vi "Log Field (No Objects).vi"(8 "error in (no error)":errorcluster, 11 "Cluster In":T4={"Field"=0.0, "Rate"=0.0, "Status"={"Sweeping"=FALSE, "Clamped"=FALSE, "Hold"=FALSE, "At Rest"=FALSE, "Quench"=FALSE, "Persistent Mode"=FALSE, "Switch Heater"=FALSE}, "ILM Shut Down?"=FALSE, "IO Info"={"Address"={"Com Port"=1, "ISOBUS Address"=2, "GPIB Address"=24, "Communication"=enum."ISOBUS"}, "Version"=enum."IPS"}, "IO Info (Level Meter)"={"Address"={"Com Port"=1, "ISOBUS Address"=5, "GPIB Address"=24, "Communication"=enum."ISOBUS"}, "ILM Name"="", "Display Channel"=[]}, "Training?"=FALSE, "Training Field and Speed Cluster"={"Training Field"=[0.0, 4.108, 5.78, 8.001], "Training Speed"=[0.0057, 0.0022833333333333334, 0.0011333333333333334, 0.0011333333333333334]}}) -> (0 "error out":errorcluster, 3 "Cluster Out":T4={"Field"=0.0, "Rate"=0.0, "Status"={"Sweeping"=FALSE, "Clamped"=FALSE, "Hold"=FALSE, "At Rest"=FALSE, "Quench"=FALSE, "Persistent Mode"=FALSE, "Switch Heater"=FALSE}, "ILM Shut Down?"=FALSE, "IO Info"={"Address"={"Com Port"=1, "ISOBUS Address"=2, "GPIB Address"=24, "Communication"=enum."ISOBUS"}, "Version"=enum."IPS"}, "IO Info (Level Meter)"={"Address"={"Com Port"=1, "ISOBUS Address"=5, "GPIB Address"=24, "Communication"=enum."ISOBUS"}, "ILM Name"="", "Display Channel"=[]}, "Training?"=FALSE, "Training Field and Speed Cluster"={"Training Field"=[0.0, 4.108, 5.78, 8.001], "Training Speed"=[0.0057, 0.0022833333333333334, 0.0011333333333333334, 0.0011333333333333334]}})   [LabVIEW 2009]
uses:
  Magnet status.ctl
  Oxford/PSSUBS.LLB/PSIO.ctl
  Oxford/BUSGEN.LLB/OxfordAddress.ctl
  Global/File Locations.vi
  Power Supply.lvclass
panel:
  out "Field":dbl[unit]
  out "status":string
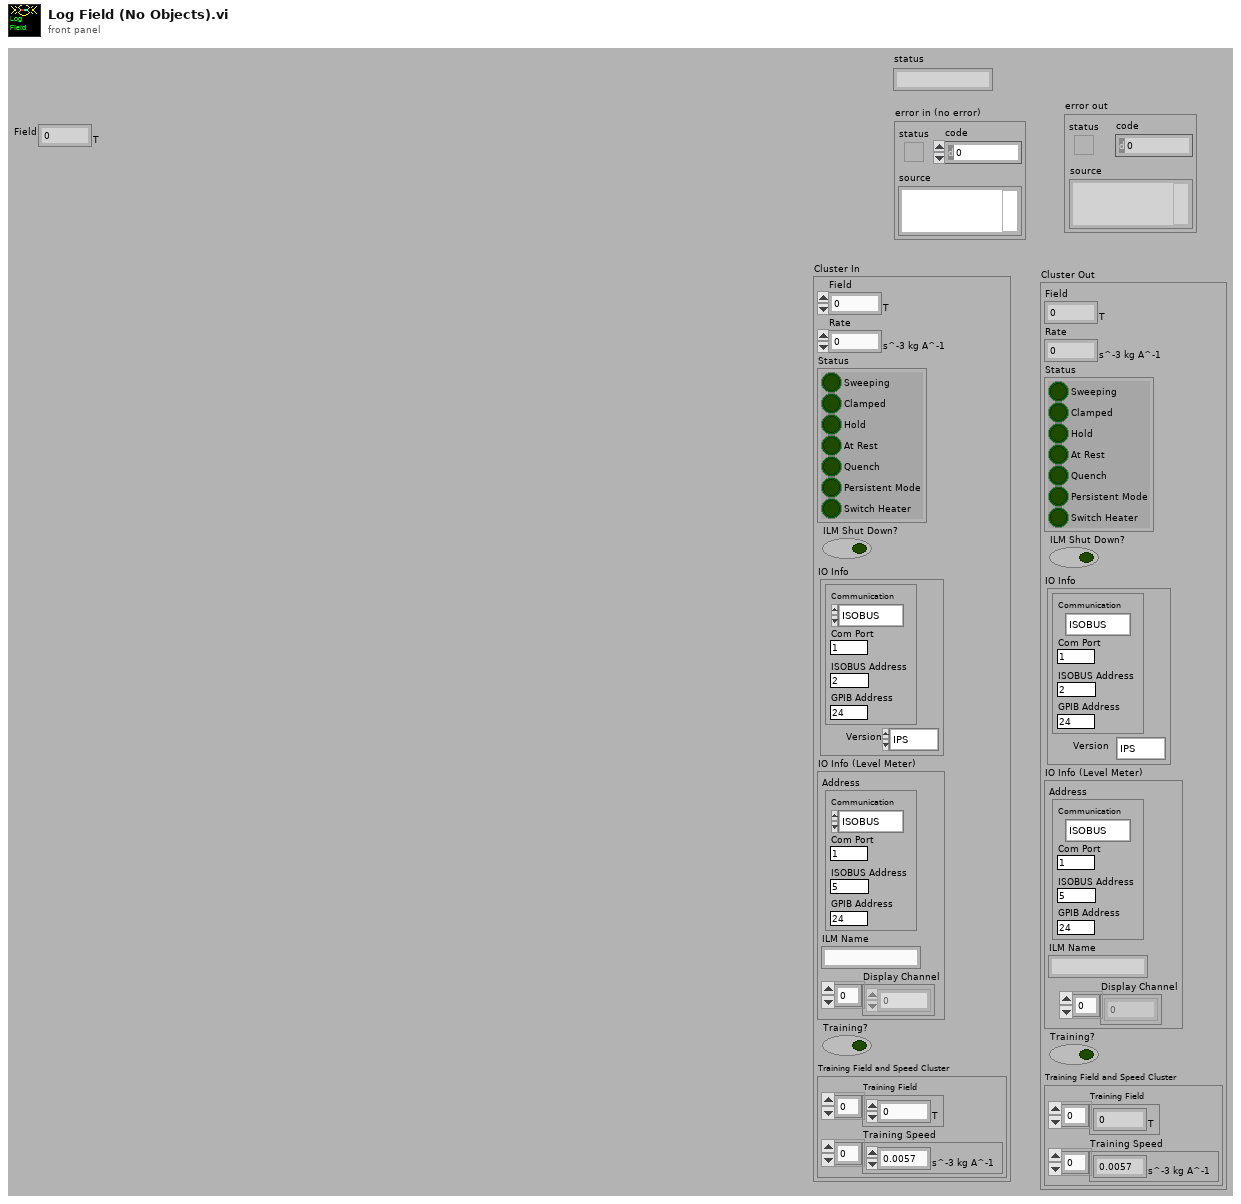
[diagram p1: front panel]
types:
  T1 = typedef "Power Supply.lvclass/Magnet status.ctl" = cluster{"Sweeping":bool, "Clamped":bool, "Hold":bool, "At Rest":bool, "Quench":bool, "Persistent Mode":bool, "Switch Heater":bool}
  T2 = typedef "PSIO.ctl" = cluster{"Address":T3, "Version":enum16{"PS", "IPS"}}
  T3 = typedef "OxfordAddress.ctl" = cluster{"Com Port":i32, "ISOBUS Address":i32, "GPIB Address":i16, "Communication":enum16{"RS232", "ISOBUS", "GPIB", "Gateway"}}
  T4 = cluster{"Field":dbl[unit], "Rate":dbl[unit], "Status":T1, "ILM Shut Down?":bool, "IO Info":T2, "IO Info (Level Meter)":cluster{"Address":T3, "ILM Name":string, "Display Channel":i32[]}, "Training?":bool, "Training Field and Speed Cluster":cluster{"Training Field":dbl[unit][], "Training Speed":dbl[unit][]}}
  T5 = enum16{"open", "open or create", "create or replace", "create", "open (read only)"}
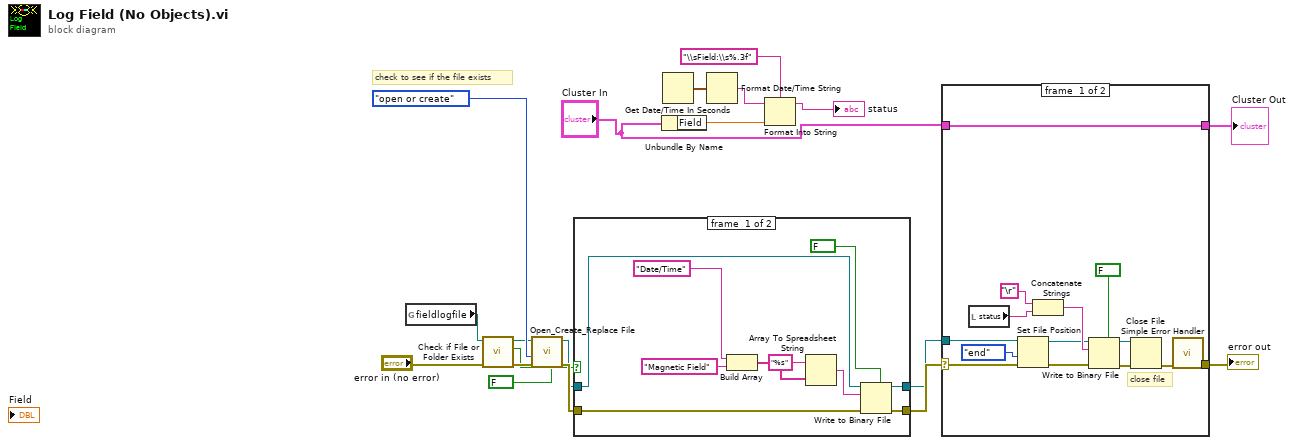
[diagram p0: block diagram]
diagram:
  # "check to see if the file exists"
  n1 = global read "File Locations.vi" "fieldlogfile"() -> (w10:path)
  n2 = call <vilib>:"Check if File or Folder Exists.vi"("error in (no error)"="error in (no error)", "path"=w10) -> ("error out"=w18:errorcluster, "file or folder exists?"=w14:bool, "dup path"=w15:path)  [unwired: 7 out]
  n3 = call <vilib>:"Open_Create_Replace File.vi"("advisory dialog? (display:T)"=FALSE, "error in (no error)"=w18, "function (open:0)"=T5."open or create", "file path"=w15) -> ("error out"=w17:errorcluster, "refnum"=w16:refnum<file>)  [unwired: 3 in, 3 out]
  n4 = case shown="False" w14 {
    tunnel: w16 -> [w29 w31]
    tunnel: w17 -> [w28 w30]
    tunnel: [w26 w31] -> w11
    tunnel: [w25 w30] -> w12
    frame #0 {
      n5 = Build Array("Date/Time", "Magnetic Field" ("element")) -> (w22:string[])
      n6 = Array To Spreadsheet String(array=w22, 3:"%s" ("format string")) -> (spreadsheet string=w21:string)  [unwired: 1 in]
      n7 = Write to Binary File(file (use dialog)=w29, data=w21, error in=w28, 5:FALSE ("prepend array or string size? (T)")) -> (refnum out=w26:refnum<file>, error out=w25:errorcluster)  [unwired: 3 out]
    }
    frame #1 {
    }
  }
  n8 = Unbundle By Name("Cluster In") -> ("Field"=w4:dbl[unit])
  n9 = Get Date/Time In Seconds() -> (seconds since 1Jan1904=w5:timestamp)
  n10 = Format Date/Time String(seconds (now)=w5) -> (date/time string=w6:string)  [unwired: 2 in]
  n11 = Format Into String(format string="\\sField:\\s%.3f", initial string=w6, w4) -> (resulting string=→"status":string)  [unwired: 1 in, 1 out]
  n12 = case shown="No Error" w12 {
    selector: w12 -> [w39 w47]
    tunnel: w11 -> [w44 _]
    tunnel: [w40 w47] -> w9
    tunnel: "Cluster In" -> [w32 w46]
    tunnel: [w32 w46] -> w1
    frame #0 {
      # "close file"
      n13 = local read "status"() -> (w36:string)
      n14 = Set File Position(refnum=w44, from (0:start)=enum16{"start", "end", "current"}."end", error in=w39) -> (refnum out=w34:refnum<file>, error out=w33:errorcluster)  [unwired: 1 out]
      n15 = Concatenate Strings("\r", w36) -> (w35:string)
      n16 = Write to Binary File(file (use dialog)=w34, data=w35, error in=w33, 5:FALSE ("prepend array or string size? (T)")) -> (refnum out=w45:refnum<file>, error out=w43:errorcluster)  [unwired: 3 out]
      n17 = Close File(refnum=w45, error in=w43) -> (error out=w42:errorcluster)  [unwired: 1 out]
      n18 = call <vilib>:"Simple Error Handler.vi"("error in (no error)"=w42) -> ("error out"=w40:errorcluster)  [unwired: 4 in, 4 out]
    }
    frame #1 {
    }
  }
  "error out" <- w9
  "Cluster Out" <- w1
